vi "E517_Wavegen_Caller.vi"(0 "System no.":i32=1 min=1 step=1, 1 "# Wavegenerators":i32, 2 "Programmatic events":T1(array[ring]), 3 "FastAxisLength":dbl, 5 "error in":errorcluster, 6 "Enabled":bool[](array[boolean])=[FALSE, FALSE, FALSE, FALSE, FALSE, FALSE, FALSE, FALSE], 7 "# WG cycles":i32[](array[numeric]) format="%#.0f", 8 "N":i32=1000, 9 "SIN_P parameters":cluster{"C":dbl, "A":dbl, "O":dbl}={"C"=500.0, "A"=5.0, "O"=0.0} {"O" format="%.6f"; "A" format="%.6f"; "C" format="%.6f"}, 10 "Xo":i32=1, 11 "TriggerVal":i32[](array[numeric])=[0, 1, 2, 4, 5, 6, 8, 9, 10, 11, 12, 14, 15, 16, 18, 19, 20, 21, 22, 24, 25, 26, 28, 29, 30, 31, 32, 34, 35, 36, 38, 39, 40, 41, 42, 44, 45, 46, 48, 49, 50, 51, 52, 54, 55, 56, 58, 59, 60, 61, 62, 64, 65, 66, 68, 69, 70, 71, 72, 74, 75, 76, 78, 79, 80, 81, 82, 84, 85, 86, 88, 89, 90, 91, 92, 94, 95, 96, 98, 99, 100, 101, 102, 104, 105, 106, 108, 109, 110, 111, 112, 114, 115, 116, 118, 119, 120, 121, 122, 124, 125, 126, 128, 129, 130, 131, 132, 134, 135, 136, 138, 139, 140, 141, 142, 144, 145, 146, 148, 149, 150, 151, 152, 154, 155, 156, 158, 159, 160, 161, 162, 164, 165, 166, 168, 169, 170, 171, 172, 174, 175, 176, 178, 179, 180, 181, 182, 184, 185, 186, 188, 189, 190, 191, 192, 194, 195, 196, 198, 199, 200, 201, 202, 204, 205, 206, 208, 209, 210, 211, 212, 214, 215, 216, 218, 219, 220, 221, 222, 224, 225, 226, 228, 229, 230, 231, 232, 234, 235, 236, 238, 239, 240, 241, 242, 244, 245, 246, 248, 249, 250, 251, 252, 254, 255, 256, 258, 259, 260, 261, 262, 264, 265, 266, 268, 269, 270, 271, 272, 274, 275, 276, 278, 279, 280, 281, 282, 284, 285, 286, 288, 289, 290, 291, 292, 294, 295, 296, 298, 299, 300, 301, 302, 304, 305, 306, 308, 309, 310, 311, 312, 314, 315, 316, 318, 319, 320, 321, 322, 324, 325, 326, 328, 329, 330, 331, 332, 334, 335, 336, 338, 339, 340, 341, 342, 344, 345, 346, 348, 349, 350, 351, 352, 354, 355, 356, 358, 359, 360, 361, 362, 364, 365, 366, 368, 369, 370, 371, 372, 374, 375, 376, 378, 379, 380, 381, 382, 384, 385, 386, 388, 389, 390, 391, 392, 394, 395, 396, 398, 399, 400, 401, 402, 404, 405, 406, 408, 409, 410, 411, 412, 414, 415, 416, 418, 419, 420, 421, 422, 424, 425, 426, 428, 429, 430, 431, 432, 434, 435, 436, 438, 439, 440, 441, 442, 444, 445, 446, 448, 449, 450, 451, 452, 454, 455, 456, 458, 459, 460, 461, 462, 464, 465, 466, 468, 469, 470, 471, 472, 474, 475, 476, 478, 479, 480, 481, 482, 484, 485, 486, 488, 489, 490, 491, 492, 494, 495, 496, 498, 499, 500, 501, 502, 504, 505, 506, 508, 509, 510, 511, 512, 514, 515, 516, 518, 519, 520, 521, 522, 524, 525, 526, 528, 529, 530, 531, 532, 534, 535, 536, 538, 539, 540, 541, 542, 544, 545, 546, 548, 549, 550, 551, 552, 554, 555, 556, 558, 559, 560, 561, 562, 564, 565, 566, 568, 569, 570, 571, 572, 574, 575, 576, 578, 579, 580, 581, 582, 584, 585, 586, 588, 589, 590, 591, 592, 594, 595, 596, 598, 599, 600, 601, 602, 604, 605, 606, 608, 609, 610, 611, 612, 614, 615, 616, 618, 619, 620, 621, 622, 624], 12 "Segm.Length":i32=1000, 13 "Append?":bool, 14 "Wavepoint":i32[](array[numeric]), 15 "Switch":i32[](array[numeric])=[0, 1, 2, 4, 5, 6, 8, 9, 10, 11, 12, 14, 15, 16, 18, 19, 20, 21, 22, 24, 25, 26, 28, 29, 30, 31, 32, 34, 35, 36, 38, 39, 40, 41, 42, 44, 45, 46, 48, 49, 50, 51, 52, 54, 55, 56, 58, 59, 60, 61, 62, 64, 65, 66, 68, 69, 70, 71, 72, 74, 75, 76, 78, 79, 80, 81, 82, 84, 85, 86, 88, 89, 90, 91, 92, 94, 95, 96, 98, 99, 100, 101, 102, 104, 105, 106, 108, 109, 110, 111, 112, 114, 115, 116, 118, 119, 120, 121, 122, 124, 125, 126, 128, 129, 130, 131, 132, 134, 135, 136, 138, 139, 140, 141, 142, 144, 145, 146, 148, 149, 150, 151, 152, 154, 155, 156, 158, 159, 160, 161, 162, 164, 165, 166, 168, 169, 170, 171, 172, 174, 175, 176, 178, 179, 180, 181, 182, 184, 185, 186, 188, 189, 190, 191, 192, 194, 195, 196, 198, 199, 200, 201, 202, 204, 205, 206, 208, 209, 210, 211, 212, 214, 215, 216, 218, 219, 220, 221, 222, 224, 225, 226, 228, 229, 230, 231, 232, 234, 235, 236, 238, 239, 240, 241, 242, 244, 245, 246, 248, 249, 250, 251, 252, 254, 255, 256, 258, 259, 260, 261, 262, 264, 265, 266, 268, 269, 270, 271, 272, 274, 275, 276, 278, 279, 280, 281, 282, 284, 285, 286, 288, 289, 290, 291, 292, 294, 295, 296, 298, 299, 300, 301, 302, 304, 305, 306, 308, 309, 310, 311, 312, 314, 315, 316, 318, 319, 320, 321, 322, 324, 325, 326, 328, 329, 330, 331, 332, 334, 335, 336, 338, 339, 340, 341, 342, 344, 345, 346, 348, 349, 350, 351, 352, 354, 355, 356, 358, 359, 360, 361, 362, 364, 365, 366, 368, 369, 370, 371, 372, 374, 375, 376, 378, 379, 380, 381, 382, 384, 385, 386, 388, 389, 390, 391, 392, 394, 395, 396, 398, 399, 400, 401, 402, 404, 405, 406, 408, 409, 410, 411, 412, 414, 415, 416, 418, 419, 420, 421, 422, 424, 425, 426, 428, 429, 430, 431, 432, 434, 435, 436, 438, 439, 440, 441, 442, 444, 445, 446, 448, 449, 450, 451, 452, 454, 455, 456, 458, 459, 460, 461, 462, 464, 465, 466, 468, 469, 470, 471, 472, 474, 475, 476, 478, 479, 480, 481, 482, 484, 485, 486, 488, 489, 490, 491, 492, 494, 495, 496, 498, 499, 500, 501, 502, 504, 505, 506, 508, 509, 510, 511, 512, 514, 515, 516, 518, 519, 520, 521, 522, 524, 525, 526, 528, 529, 530, 531, 532, 534, 535, 536, 538, 539, 540, 541, 542, 544, 545, 546, 548, 549, 550, 551, 552, 554, 555, 556, 558, 559, 560, 561, 562, 564, 565, 566, 568, 569, 570, 571, 572, 574, 575, 576, 578, 579, 580, 581, 582, 584, 585, 586, 588, 589, 590, 591, 592, 594, 595, 596, 598, 599, 600, 601, 602, 604, 605, 606, 608, 609, 610, 611, 612, 614, 615, 616, 618, 619, 620, 621, 622, 624]) -> (16 "Triggerpoints":dbl[][](graph), 17 "Wavetable data":dbl[][](graph), 18 "Recordtable data":dbl[][](graph), 19 "Error out":errorcluster)   [LabVIEW 2011]
doc: "This VI demonstrates how to configure the wave generator, set wave tables, read data recorder tables and set trigger points. The diagram shows how to combine the driver VIs for these tasks. \nThe controls connected to the connector pane exemplify the application. You can modify the connector pane and add controls to meet your requirements. The E517_Wavegen_Example_Caller.vi shows how to call this VI programmatically as a SubVI.\n\nRun E517_Configuration_Setup.vi prior to running this VI.\n\nOn the [Settings] tab you can link wave tables to wave generators if this feature is supported by your controller, adjust wave table and record table rates and configure the wave generator. The current wave generator mode setting (WGO), the actual positions and the servo states are updated continuously.\n \nSelect the desired wave table on the [Wavetables] tab to write a waveform into it or to clean a previously stored waveform. #points in WT shows the actual length of the tables. You can apply controller generated sine waves or host PC generated point-by-point ramp waveforms covering the motion range of the appropriate connected stage. Please consult the Context Help window of the WAV.vi the User Manual of your controller for details on waveform settings. After writing a waveform to the controller all waveforms are read back and displayed automatically. You can read out the wave tables manually, too.\n\nAll further tabs are disabled until you have defined one wave table at least.\n \nConfigure the data recorder on the [Recordtables] tab prior to reading out any data. Each data recorder table must be configured separately by choosing a linked axis and an axis related record option. The contents of the data recorder tables are not read out automatically. Reasonable data is only available if at least one wave generator run has been started since the last power-on / reboot of the controller.\n \nOn the [Triggerpoints] tab you can link axes to triggerlines if this feature is supported by your controller. If you want to output trigger pulses synchronized with the wave generator output, activate the Generator Trigger mode by pressing the Set TWS trigger mode button. The trigger related controls will then be activated. In the matrix you can define the active trigger points for each triggerline. They will be written to the controller's RAM by Set these trigger points. To reset trigger points use Clear all trigger points. In the graphics pane the active trigger points are displayed as bars."
panel:
  in  "LIN Parameters":cluster{"J":dbl, "A":dbl, "O":dbl}={"J"=0.0, "A"=10.0, "O"=0.0}
  out "Number of Triggerlines":i32
  out "SubVI":bool
  out "Running?":bool[](array[boolean])
  in  "Tab Control":T2(tab)
  out "Axes":string[](array[string])
  in  "Recordtable rate":i32=1
  in  "Wavegen":i32[](array[numeric])=[1, 2, 3] format="%#.0f"
  out "# Recordtables":i32
  out "# Wavetables":i32
  out "# Wavegenerators":i32
  out "Servo":bool[](array[boolean])
  in  "Wavetable rate":i32[](array[numeric]) format="%#.0f"
  out "Positions":dbl[](array[numeric])
  out "WGO mode":i32[](array[numeric]) format="%#.0f"
  in  "Start at\nEndpoint":bool[](array[boolean])=[FALSE, FALSE, FALSE, FALSE, FALSE, FALSE, FALSE, FALSE]
  in  "DDL init":bool[](array[boolean])=[FALSE, FALSE, FALSE, FALSE, FALSE, FALSE, FALSE, FALSE]
  in  "DDL enable":bool[](array[boolean])=[FALSE, FALSE, FALSE, FALSE, FALSE, FALSE, FALSE, FALSE]
  in  "GWD?":bool
  out "# points in WT":i32[](array[numeric]) format="%#.0f"
  in  "WCL":bool
  in  "Write sine":bool
  in  "Add?":bool
  in  "Write points":bool
  out "Assigned\nwavegenerator":i32
  in  "Wavetable":u16(ring) items=["1"]
  in  "DRC?":bool
  out "Record option":string[](array[string])
  out "Source ID":string[](array[string])
  in  "DRC":bool
  in  "Record option":u16(ring)=1 items=["Target position of axis "=1, "Current position of axis "=2, "Position error of axis "=3, "Voltage of piezo channel "=7, "Control output of axis "=15, "DAC input of piezo channel "=16]
  in  "Axis":u16(ring) items=["1"]
  in  "Record table":u16(ring) items=["1", "2", "3"]
  in  "N:":i32=1000
  in  "X0:":i32=1
  in  "DRR?":bool
  in  "CTO":bool
  in  "TWC":bool
  in  "TWS":bool
  in  "TWS?":bool
  in  "Axis":u16[](array[ring]) items=["1"]
  in  "Clear error":bool
  in  "Stop":bool
  # "E-517 wave generator, data recorder and trigger setting sample program"
  # "This VI demonstrates how to configure the wave generator, set wavetables, read recordtables and set triggerpoints.\nYou can apply controller generated sine waves or host PC generated point-by-point ramp waveforms.\nRun E517_Configuration_Setup.vi prior to running this VI."
  # "Wavegenerator state:"
  # "Wavetable"
  # "1"
  # "2"
  # "3"
  # "4"
  # "5"
  # "6"
  # "7"
  # "8"
  # "Wavegen"
  # "1"
  # "2"
  # "3"
  # "4"
  # "5"
  # "6"
  # "7"
  # "8"
  # "1"
  # "2"
  # "3"
  # "4"
  # "5"
  # "6"
  # "7"
  # "8"
  # "1black 2red 3green 4cyan 5yelllow 6purple 7orange 8blue"
  # "1"
  # "2"
  # "3"
  # "4"
  # "5"
  # "6"
  # "7"
  # "8"
  # "1black 2red 3green 4cyan 5yelllow 6purple 7orange 8blue"
  # "Trigger"
  # "1"
  # "2"
  # "3"
  # "4"
  # "5"
  # "6"
  # "1black 2red 3green 4blue 5yelllow 6purple"
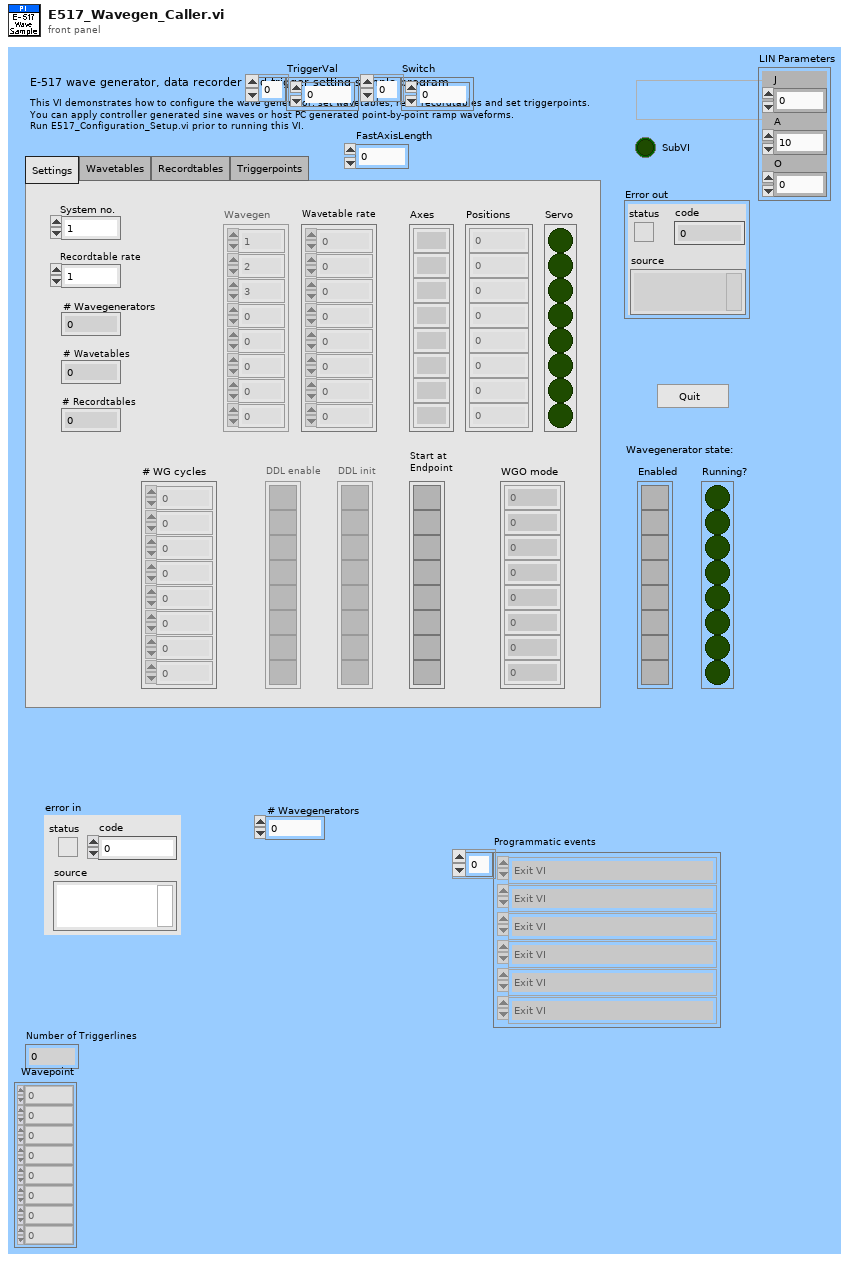
[diagram p1: front panel]
types:
  T1 = enum16{"Exit VI", "Set trigger mode", "Set recordtable rate", "Set wavetable rate", "Write sine", "Read wavetable", "Read recordtable", "Enable/disable wavegen", "Set number of wavegen cycles", "Clear wavetable", "Configure data recorder", "Assign wavetable to wavegen", "Read trigger points", "Set trigger points", "Clear trigger points", "Assign axes to triggerlines", "Write ramp waveform", "Set DDL enable", "Set DDL init", "Set Start at endpoint"}[]
  T2 = enum32{"Settings", "Wavetables", "Recordtables", "Triggerpoints"}
  T3 = enum32{"Page Enabled", "Page Disabled", "Page Disabled & Grayed"}
  T4 = enum16{"Position Distance", "Position Distance & Wait Time", "OnTarget", "MinMax Threshold", "Generator Trigger (TWS)", "Motion Error", "In Motion"}
  T5 = enum16{"Unused", "TriggerStep", "Axis", "TriggerMode", "TriggerDelay", "MinThreshold", "MaxThreshold", "Polarity", "StartThreshold", "StopThreshold"}
  T6 = enum16{"Position Distance", "Position Distance & Wait Time", "OnTarget", "MinMax Threshold", "Generator Trigger (TWS)", "Motion Error", "In Motion"}[]
  T7 = enum16{"Unused", "TriggerStep", "Axis", "TriggerMode", "TriggerDelay", "MinThreshold", "MaxThreshold", "Polarity", "StartThreshold", "StopThreshold"}[]
  T8 = enum16{"Exit VI", "Set trigger mode", "Set recordtable rate", "Set wavetable rate", "Write sine", "Read wavetable", "Read recordtable", "Enable/disable wavegen", "Set number of wavegen cycles", "Clear wavetable", "Configure data recorder", "Assign wavetable to wavegen", "Read trigger points", "Set trigger points", "Clear trigger points", "Assign axes to triggerlines", "Write ramp waveform", "Set DDL enable", "Set DDL init", "Set Start at endpoint"}
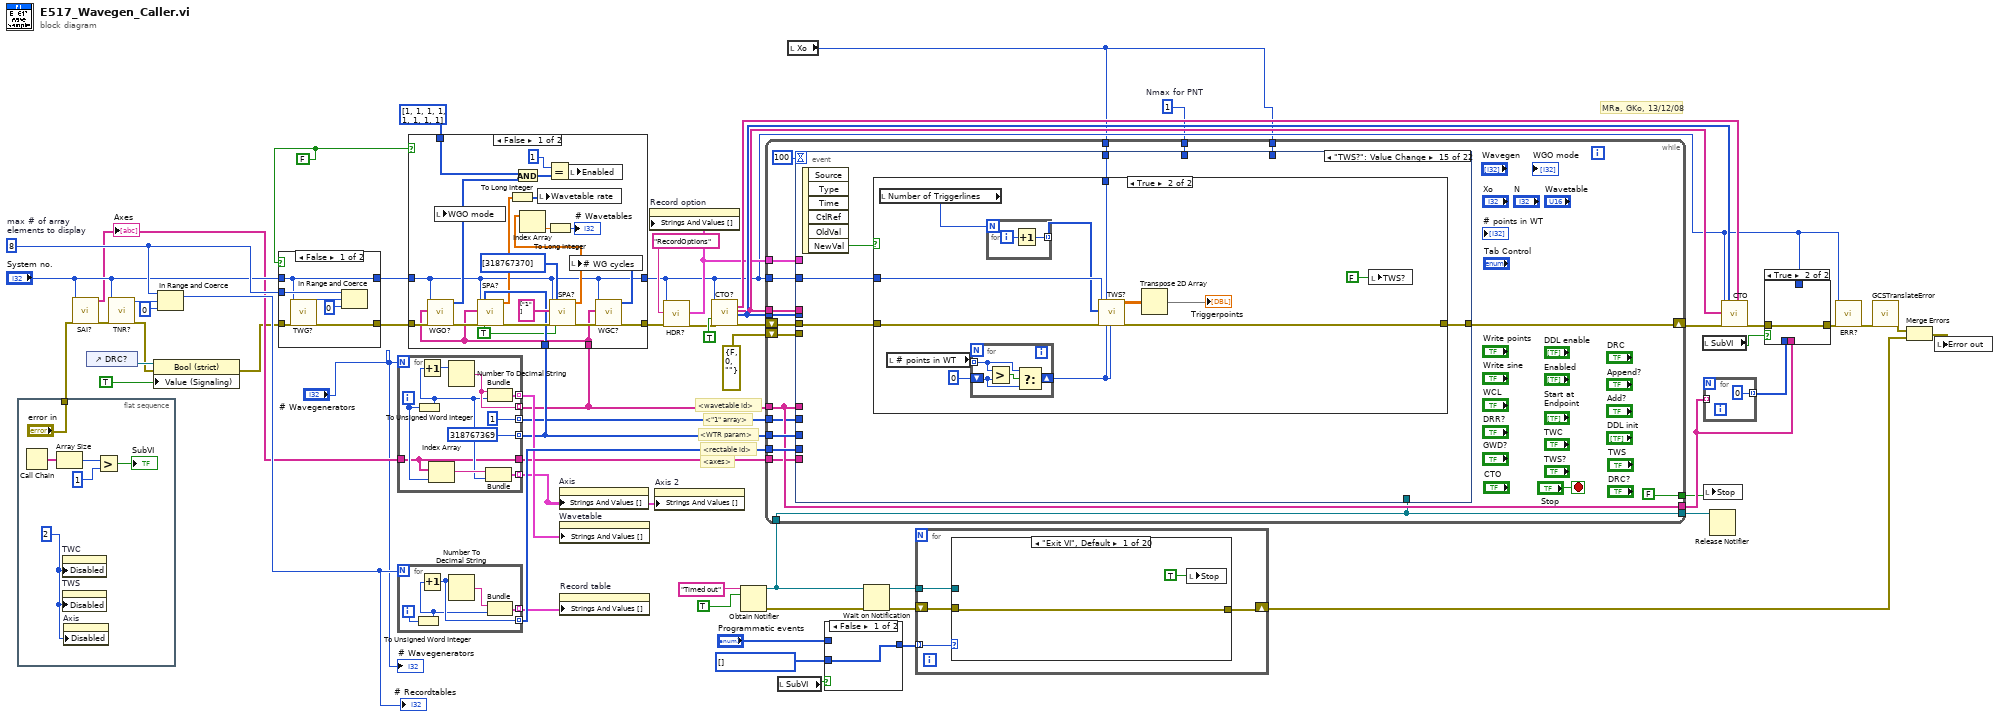
[diagram p0: block diagram]
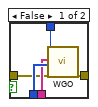
[diagram p2: hidden frame]
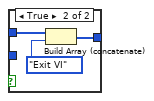
[diagram p5: hidden frame]
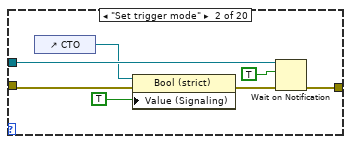
[diagram p6: hidden frame]
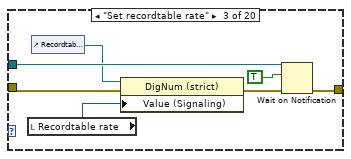
[diagram p7: hidden frame]
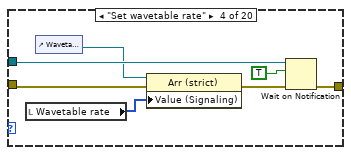
[diagram p8: hidden frame]
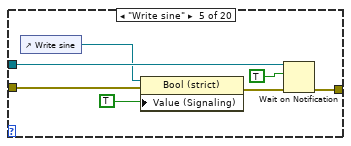
[diagram p9: hidden frame]
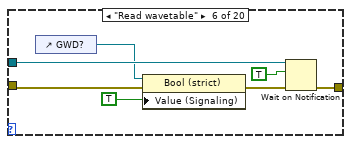
[diagram p10: hidden frame]
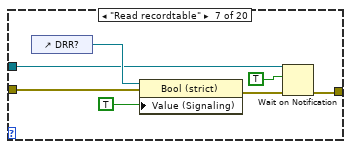
[diagram p11: hidden frame]
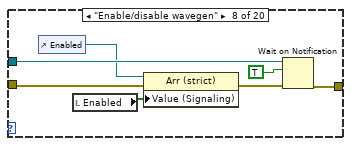
[diagram p12: hidden frame]
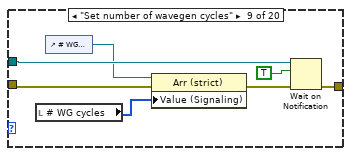
[diagram p13: hidden frame]
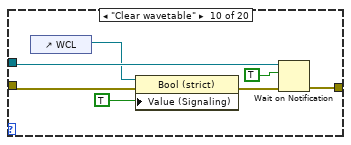
[diagram p14: hidden frame]
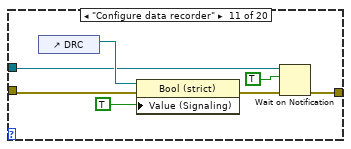
[diagram p15: hidden frame]
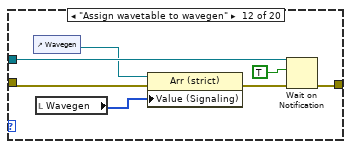
[diagram p16: hidden frame]
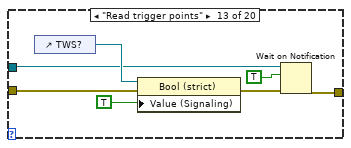
[diagram p17: hidden frame]
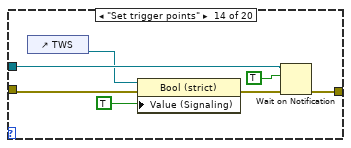
[diagram p18: hidden frame]
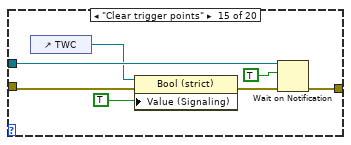
[diagram p19: hidden frame]
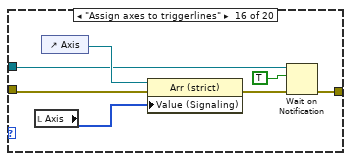
[diagram p20: hidden frame]
diagram:
  w1 = FALSE
  w16 = T1 [] items=["Exit VI", "Set trigger mode", "Set recordtable rate", "Set wavetable rate", "Write sine", "Read wavetable", "Read recordtable", "Enable/disable wavegen", "Set number of wavegen cycles", "Clear wavetable", "Configure data recorder", "Assign wavetable to wavegen", "Read trigger points", "Set trigger points", "Clear trigger points", "Assign axes to triggerlines", "Write ramp waveform", "Set DDL enable", "Set DDL init", "Set Start at endpoint"] ("Programmatic events")
  w4 = 1  # Nmax for PNT
  w13 = 8  # max # of array  elements to display
  # "<axes>"
  # "MRa, GKo, 13/12/08"
  # "<wavetable id>"
  # "<rectable id>"
  # "<\"1\" array>"
  # "<WTR param>"
  n1 = flat-sequence {
    tunnel: ["error in"] -> w20
    frame #0 {
      w61 = u8 2 ("Disabled")
      n2 = Call Chain() -> (call chain=w66:string[])
      n3 = Array Size(array=w66) -> (size(s)=w65:i32)
      n4 = property on="TWC" class="Bool (strict)"("Disabled"=w61) -> ()  [unwired: 2 in, 2 out]
      n5 = property on="TWS" class="Bool (strict)"("Disabled"=w61) -> ()  [unwired: 2 in, 2 out]
      n6 = property on="Axis" class="Arr (strict)"("Disabled"=w61) -> ()  [unwired: 2 in, 2 out]
      n7 = Greater?(x=w65, y=1) -> (0:→"SubVI":bool)
    }
  }
  n8 = call "SAI?.vi"("System no."="System no.", "error in"=w20) -> ("Conn. axes"=w8:string[], "error out"=w51:errorcluster)  [unwired: 3 in, 13 out]
  "Axes" <- w8
  n9 = control-ref of="DRC?"() -> (w48:refnum<vi>)
  n10 = call "TNR?.vi"("System no."="System no.", "error in"=w51) -> ("Number of Rec. tables"=w56:i32, "error out"=w15:errorcluster)  [unwired: 16 out]
  n11 = property class="Bool (strict)"(reference=w48, error in=w15, "Value (Signaling)"=TRUE ("TWC")) -> (error out=w6:errorcluster)  [unwired: 1 out]
  n12 = In Range and Coerce(upper limit=w13, x=w56, lower limit=0) -> (coerced(x)=w10:i32)  [unwired: 1 out]
  "# Recordtables" <- w10
  n13 = case shown="False" w1 {
    tunnel: [w72 w73] -> w14
    tunnel: w6 -> [w71 w73]
    tunnel: w13 -> [w69 _]
    tunnel: "System no." -> [w67 w74]
    tunnel: [w67 w74] -> w11
    frame False {
      n14 = call "TWG?.vi"("System no."=w67, "error in"=w71) -> ("Number of wave generators"=w70:i32, "error out"=w72:errorcluster)  [unwired: 16 out]
      n15 = In Range and Coerce(upper limit=w69, x=w70, lower limit=0) -> ()  [unwired: 2 out]
    }
    frame True {
    }
  }
  n16 = for {
    N: "# Wavegenerators" -> [_]
    tunnel: [w83] -> w58 mode=indexing
    tunnel: [w78] -> w19 mode=indexing
    tunnel: [318767369 ("Numeric")] -> w55 mode=indexing
    tunnel: [1 ("Number of wave generators")] -> w50 mode=indexing
    tunnel: w8 -> [w75]
    tunnel: [w77] -> w5 mode=indexing
    tunnel: [w75] -> w7
    i -> [w80]
    n17 = To Unsigned Word Integer(number=w80) -> (unsigned 16bit integer=w76:u16)
    n18 = Increment(x=w76) -> (x+1=w84:u16)
    n19 = Index Array(array=w75, index=w80) -> (element=w79:string)
    n20 = Number To Decimal String(number=w84) -> (decimal integer string=w78:string)  [unwired: 1 out]
    n21 = Bundle("String"=w79, w76) -> (w77:cluster{"String":string, u16})  [unwired: 1 out]
    n22 = Bundle(w78, w76) -> (w83:cluster{string, u16})  [unwired: 1 out]
  }
  n23 = for {
    N: w10 -> [_]
    tunnel: [w89] -> w59 mode=indexing
    tunnel: [w87] -> w60 mode=indexing
    i -> [w86]
    n24 = To Unsigned Word Integer(number=w86) -> (unsigned 16bit integer=w85:u16)
    n25 = Increment(x=w85) -> (x+1=w87:u16)
    n26 = Number To Decimal String(number=w87) -> (decimal integer string=w88:string)  [unwired: 1 out]
    n27 = Bundle(w88, w85) -> (w89:cluster{string, u16})  [unwired: 1 out]
  }
  n28 = case shown="False" w1 {
    tunnel: w14 -> [w111 w112]
    tunnel: w55 -> [w106 _]
    tunnel: [w105 w112] -> w26
    tunnel: w11 -> [w91 w113]
    tunnel: i32[] [1, 1, 1, 1, 1, 1, 1, 1] ("WGO parameter") -> [w101 _]
    tunnel: [w91 w113] -> w21
    tunnel: w19 -> [w90 _]
    frame False {
      w94 = TRUE ("Parameter no. format \n(Decimal: FALSE)")
      n29 = call "WGO?.vi"("System no."=w91, "Axes to query"=w90, "error in"=w111) -> ("WGO parameter"=w100:i32[], "error out"=w108:errorcluster)  [unwired: 2 in, 13 out]
      n30 = local write "WGO mode"(w100) -> ()
      n31 = call "SPA?.vi"("System no."=w91, "Axes to query"=w90, "error in"=w108, "Parameter no. (hex)"=w106, "Parameter no. format \n(Decimal: FALSE)"=w94) -> ("Parameter value"=w98:dbl[], "error out"=w107:errorcluster)  [unwired: 2 in, 11 out]
      n32 = To Long Integer(number=w98) -> (32bit integer=w99:i32[])
      n33 = And(x=w101, y=w100) -> (x .and. y?=w102:i32[])
      n34 = local write "Wavetable rate"(w99) -> ()
      n35 = Equal?(x=1, y=w102) -> (x = y?=w104:bool[])
      n36 = call "SPA?.vi"("System no."=w91, "Axes to query"=string[] ["1"], "error in"=w107, "Parameter no. (hex)"=u32[] [318767370], "Parameter no. format \n(Decimal: FALSE)"=w94) -> ("Parameter value"=w92:dbl[], "error out"=w110:errorcluster)  [unwired: 2 in, 11 out]
      n37 = Index Array(array=w92) -> (element=w97:dbl)  [unwired: 1 in]
      n38 = To Long Integer(number=w97) -> (32bit integer=→"# Wavetables":i32)
      n39 = local write "Enabled"(w104) -> ()
      n40 = call "WGC?.vi"("System no."=w91, "Axes to query"=w90, "error in"=w110) -> ("Cycles"=w95:i32[], "error out"=w105:errorcluster)  [unwired: 2 in, 13 out]
      n41 = local write "# WG cycles"(w95) -> ()
    }
    frame True {
    }
  }
  n42 = property on="Axis" class="Ring (strict)"("Strings And Values []"=w5) -> ()  [unwired: 2 in, 2 out]
  n43 = property on="Wavetable" class="Ring (strict)"("Strings And Values []"=w58) -> ()  [unwired: 2 in, 2 out]
  n44 = property on="Record table" class="Ring (strict)"("Strings And Values []"=w59) -> ()  [unwired: 2 in, 2 out]
  n45 = property on="Axis 2" class="Ring (strict)"("Strings And Values []"=w5) -> ()  [unwired: 2 in, 2 out]
  n46 = call "HDR?.vi"("System no."=w21, "Section header"="RecordOptions" ("Header"), "error in"=w26) -> ("Enum values"=w23:cluster{"token string":string, i32}[], "error out"=w25:errorcluster)  [unwired: 15 out]
  n47 = property on="Record option" class="Ring (strict)"("Strings And Values []"=w23) -> ()  [unwired: 2 in, 2 out]
  n48 = call "CTO?.vi"("System no."=w21, "All Triggers?"=TRUE, "error in"=w25) -> ("Parameter value"=w41:string[], "TriggerOut to query out"=w39:string[], "CTO parameter ID out"=w40:i32[], "error out"=w47:errorcluster)  [unwired: 2 in, 11 out]
  n49 = Obtain Notifier(name (unnamed)="Timed out", notification data type=TRUE ("GWD?")) -> (notifier out=w30:refnum<notifier>, error out=w33:errorcluster)  [unwired: 2 in, 1 out]
  n50 = local read "SubVI"() -> (w18:bool)
  n51 = local read "Xo"() -> (w3:i32)
  n52 = while {
    tunnel: w21 -> [w123]
    shift-right: [w127] -> w43
    shift-left: w47 -> [w131]
    tunnel: w19 -> [w125]
    tunnel: w60 -> [w129]
    tunnel: w23 -> [w128]
    tunnel: w55 -> [w126]
    tunnel: [w125] -> w44
    shift-left: errorcluster {"status"=FALSE, "code"=0, "source"=""} ("error in") -> [w124]
    tunnel: w50 -> [w122]
    tunnel: w3 -> [w121]
    tunnel: w3 -> [w120]
    tunnel: w4 -> [w119]
    tunnel: w40 -> [w118]
    tunnel: w39 -> [w117]
    tunnel: [FALSE ("Stop")] -> w37
    tunnel: [w115] -> w34
    tunnel: w30 -> [w115]
    tunnel: w7 -> [w114]
    stop <- "Stop" stop-if-true
    n53 = event shown="[14] \"TWS?\": Value Change" {
      selector: _ -> [_ _ _ _ _ _ _ _ _ _ _ _ _ _ _ _ _ _ _ _ _ _]
      dyn-events: _ -> [_ _ _ _ _ _ _ _ _ _ _ _ _ _ _ _ _ _ _ _ _ _]
      timeout: 100 -> [_ _ _ _ _ _ _ _ _ _ _ _ _ _ _ _ _ _ _ _ _ _]
      tunnel: w131 -> [w140 w187 w219 w227 w230 w260 w265 w301 w330 w335 w338 w362 w386 w412 w416 w440 w469 w483 w504 w535 w544 w553]
      tunnel: w123 -> [w144 w185 w217 w223 w229 _ w264 w300 w321 w334 w337 w361 w385 _ w415 w439 w467 w486 w503 _ _ _]
      tunnel: w125 -> [_ _ _ w222 w231 _ w266 w302 w320 w333 w339 _ w387 _ _ _ _ _ w502 _ _ _]
      tunnel: w129 -> [_ _ _ _ _ _ _ w299 _ _ _ w360 _ _ _ _ _ _ _ _ _ _]
      tunnel: w128 -> [_ _ _ _ _ _ _ _ _ _ _ w359 w384 _ _ _ _ _ _ _ _ _]
      tunnel: [w141 w186 w218 w226 w228 w260 w263 w298 w322 w331 w336 w358 w383 w412 w414 w438 w468 w484 w500 w535 w544 w553] -> w127
      tunnel: w126 -> [_ _ _ w221 _ _ _ _ _ _ _ _ _ _ _ _ _ _ _ _ _ _]
      tunnel: w124 -> [w139 _ _ _ _ _ _ _ _ _ _ _ _ _ _ _ _ _ _ _ _ _]
      tunnel: w122 -> [_ _ _ _ _ _ w262 _ _ _ _ _ _ _ _ _ _ _ _ _ _ _]
      tunnel: w121 -> [_ _ _ _ _ _ w261 _ _ _ _ _ _ _ _ _ _ _ _ _ _ _]
      tunnel: w120 -> [_ _ _ _ _ _ _ _ _ _ _ _ _ _ w413 _ _ _ _ _ _ _]
      tunnel: w119 -> [_ _ _ _ _ _ _ _ _ _ _ _ _ _ _ _ _ _ w499 _ _ _]
      tunnel: w118 -> [_ w184 _ _ _ _ _ _ _ _ _ _ _ _ _ _ _ _ _ _ _ _]
      tunnel: w117 -> [_ w183 _ _ _ _ _ _ _ _ _ _ _ _ _ _ _ _ _ _ _ _]
      tunnel: w115 -> [w133 _ _ _ _ _ _ _ _ _ _ _ _ _ _ _ _ _ _ _ _ _]
      tunnel: w114 -> [_ _ _ _ _ _ _ _ _ _ _ w357 _ _ _ _ _ w490 _ _ _ _]
      event Timeout {
        n54 = event-data() -> ()  [unwired: 3 out]
        n55 = Unbundle By Name(w139) -> ("status"=w137:bool)
        n56 = call "ERR?.vi"("System no."=w144, "error in"=w140) -> ("error out"=w135:errorcluster)  [unwired: 17 out]
        n57 = Unbundle By Name(w135) -> ("status"=w138:bool)
        n58 = Not Equal?(x=w138, y=w137) -> (x != y?=w136:bool)
        n59 = case shown="False" w136 {
          tunnel: w135 -> [w145 w147]
          tunnel: [w145 w146] -> w143
          frame False {
          }
          frame True {
            n60 = call "GCSTranslateError.vi"("error in"=w147) -> ("error out"=w146:errorcluster)  [unwired: 18 out]
          }
        }
        n61 = case shown="No Error" w143 {
          selector: w143 -> [w148 w178]
          tunnel: [w149 w179] -> w141
          tunnel: w144 -> [w161 _]
          frame No Error {
            w151 = TRUE  # All axes?
            n62 = local read "# points in WT"() -> (w155:i32[])
            n63 = Greater Than 0?(x=w155) -> (x > 0?=w154:bool[])
            n64 = Or Array Elements(Boolean array=w154) -> (logical OR=w156:bool)
            n65 = call "#9.vi"("System no."=w161, "error in"=w148) -> ("WG running?"=→"Running?":bool[], "error out"=w164:errorcluster)  [unwired: 16 out]
            n66 = Select(t=T3."Page Enabled" ("Page Enabled State"), s=w156, f=T3."Page Disabled & Grayed" ("Page Enabled State")) -> (s? t:f=w159:T3)
            n67 = call "POS?.vi"("System no."=w161, "All axes?"=w151, "error in"=w164) -> ("Position"=→"Positions":dbl[], "error out"=w162:errorcluster)  [unwired: 2 in, 13 out]
            n68 = call "SVO?.vi"("System no."=w161, "All axes?"=w151, "error in"=w162) -> ("Servo status?"=→"Servo":bool[], "error out"=w150:errorcluster)  [unwired: 2 in, 13 out]
            n69 = property on="Tab Control" class="TabCtl (strict)"(error in=w150) -> (error out=w153:errorcluster, "Pages"=w152:refnum<vi>[])  [unwired: 1 in, 1 out]
            n70 = for {
              shift-right: [w171] -> w149
              shift-left: w153 -> [w172]
              tunnel: w152 -> [w170] mode=indexing
              tunnel: w159 -> [w169]
              i -> [w168]
              n71 = Greater?(x=w168, y=1) -> (0:w166:bool)
              n72 = case shown="True" w166 {
                tunnel: w172 -> [w173 w177]
                tunnel: [w173 w176] -> w171
                tunnel: w170 -> [_ w175]
                tunnel: w169 -> [_ w174]
                frame False {
                }
                frame True {
                  n73 = property class="Page"(reference=w175, error in=w177, "Page Enabled State"=w174) -> (error out=w176:errorcluster)  [unwired: 1 out]
                }
              }
            }
          }
          frame Error {
            n74 = Select(t=errorcluster {"status"=FALSE, "code"=0, "source"=""}, s="Clear error", f=w178) -> (s? t:f=w179:errorcluster)
          }
        }
        "Error out" <- w141
        n75 = Unbundle By Name(w141) -> ("status"=w142:bool)
        n76 = property on="Clear error" class="Bool"("Visible"=w142) -> ()  [unwired: 2 in, 2 out]
        n77 = Send Notification(notification=TRUE, notifier=w133) -> ()  [unwired: 1 in, 2 out]
      }
      event "CTO": Value Change {
        n78 = event-data() -> ("NewVal"=w182:bool)  [unwired: 6 out]
        n79 = case shown="True" w182 {
          tunnel: w187 -> [w188 w205]
          tunnel: [w188 w204] -> w186
          tunnel: w185 -> [_ w203]
          tunnel: w184 -> [_ w202]
          tunnel: w183 -> [_ w201]
          frame False {
          }
          frame True {
            w190 = u8 0 ("Disabled")
            # "Not supported"
            n80 = for {
              tunnel: w202 -> [w211] mode=indexing
              tunnel: w201 -> [w207] mode=indexing
              shift-right: [w208] -> w193
              shift-left: string[] [] -> [w209]
              tunnel: T5."TriggerMode" -> [w206]
              n81 = Equal?(x=w211, y=w206) -> (x = y?=w210:bool)
              n82 = case shown="False" w210 {
                tunnel: w209 -> [w212 w215]
                tunnel: [w212 w214] -> w208
                tunnel: w207 -> [_ w213]
                frame False {
                }
                frame True {
                  n83 = Build Array (concatenate)(w215, w213) -> (w214:string[])
                }
              }
            }
            n84 = property on="TWC" class="Bool (strict)"("Disabled"=w190) -> ()  [unwired: 2 in, 2 out]
            n85 = property on="TWS" class="Bool (strict)"("Disabled"=w190) -> ()  [unwired: 2 in, 2 out]
            n86 = Array Size(array=w193) -> (size(s)=w199:i32)
            "Number of Triggerlines" <- w199
            n87 = property on="Axis" class="Arr (strict)"("Disabled"=u8 2) -> ()  [unwired: 2 in, 2 out]
            n88 = Initialize Array(T4."Generator Trigger (TWS)", w199) -> (w198:T6)
            n89 = Initialize Array(T5."TriggerMode", w199) -> (w191:T7)
            n90 = Number To Decimal String(number=w198) -> (decimal integer string=w197:string[])  [unwired: 1 out]
            n91 = call "CTO.vi"("System no."=w203, "TriggerOut to set"=w193, "error in"=w205, "CTO parameter ID"=w191, "Parameter value"=w197) -> ("error out"=w204:errorcluster)  [unwired: 1 in, 13 out]
            n92 = local write "CTO"(FALSE ("CTO")) -> ()
          }
        }
      }
      event "Recordtable rate": Value Change {
        n93 = event-data() -> ()  [unwired: 7 out]
        n94 = call "RTR.vi"("System no."=w217, "Table rate"="Recordtable rate", "error in"=w219) -> ("error out"=w218:errorcluster)  [unwired: 16 out]
      }
      event "Wavetable rate": Value Change {
        n95 = event-data() -> ()  [unwired: 7 out]
        n96 = To Double Precision Float(number="Wavetable rate") -> (double precision float=w224:dbl[])
        n97 = call "SPA.vi"("System no."=w223, "Axis to set"=w222, "Parameter value"=w224, "error in"=w227, "Parameter no. format \n(Decimal: FALSE)"=TRUE ("Parameter no. format \n(Decimal: FALSE)"), "Parameter number (hex)"=w221) -> ("error out"=w226:errorcluster)  [unwired: 4 in, 9 out]
      }
      event "Write sine": Value Change {
        n98 = event-data() -> ("NewVal"=w232:bool)  [unwired: 6 out]
        n99 = case shown="True" w232 {
          tunnel: w230 -> [w233 w236]
          tunnel: [w233 w235] -> w228
          tunnel: w229 -> [_ w240]
          tunnel: w231 -> [_ w241]
          frame False {
          }
          frame True {
            w251 = u16 4 items=["SIN", "POL", "TAN", "PNT", "SIN_P", "LIN", "RAMP"] ("Waveform")
            n100 = local read "Wavetable"() -> (w239:u16)
            n101 = local read "N"() -> (w244:i32)
            n102 = local read "Append?"() -> (w248:bool)
            n103 = local read "Xo"() -> (w246:i32)
            n104 = local read "Add?"() -> (w247:bool)
            n105 = Index Array(array=w241, index=w239) -> (element=w250:string)
            n106 = Build Array(w250) -> (w249:string[])
            n107 = call "WAV.vi"("System no."=w240, "Waveform"=w251, "Affected axes"=w249, "Append? (&)"=w248, "Add? (+)"=w247, "error in"=w236, "Xo"=w246, "N"=w244, "Segment length"="Segm.Length", "SIN_P Parameters"="SIN_P parameters") -> ("error out"=w242:errorcluster)  [unwired: 8 in, 9 out]
            n108 = call "Wait for controller ready.vi"("System no."=w240, "error in"=w242) -> ("error out"=w238:errorcluster)  [unwired: 2 in, 15 out]
            n109 = local read "SubVI"() -> (w234:bool)
            n110 = case shown="False" w234 {
              tunnel: w238 -> [w253 w256]
              tunnel: [w252 w256] -> w235
              frame False {
                n111 = control-ref of="GWD?"() -> (w255:refnum<vi>)
                n112 = property class="Bool (strict)"(reference=w255, error in=w253, "Value (Signaling)"=TRUE ("GWD?")) -> (error out=w252:errorcluster)  [unwired: 1 out]
              }
              frame True {
              }
            }
            n113 = local write "Write sine"(FALSE ("Write sine")) -> ()
          }
        }
      }
      event "Wavetable": Value Change {
        n114 = event-data() -> ("NewVal"=w259:u16)  [unwired: 6 out]
        n115 = local read "Wavegen"() -> (w258:i32[])
        n116 = Index Array(array=w258, index=w259) -> (element=→"Assigned\nwavegenerator":i32)
      }
      event "GWD?": Value Change {
        n117 = event-data() -> ("NewVal"=w267:bool)  [unwired: 6 out]
        n118 = case shown="True" w267 {
          tunnel: w265 -> [w268 w278]
          tunnel: [w268 w269] -> w263
          tunnel: w264 -> [_ w275]
          tunnel: w266 -> [_ w274]
          tunnel: w262 -> [_ w273]
          tunnel: w261 -> [_ w272]
          frame False {
          }
          frame True {
            n119 = call "WAV?.vi"("System no."=w275, "Axes to query"=w274, "Parameter no."=w273, "error in"=w278) -> ("WAV Parameter value"=w276:dbl[], "error out"=w271:errorcluster)  [unwired: 14 out]
            n120 = To Long Integer(number=w276) -> (32bit integer=w277:i32[])
            n121 = local write "# points in WT"(w277) -> ()
            n122 = for {
              tunnel: w275 -> [w285]
              tunnel: w274 -> [w284] mode=indexing
              tunnel: [w283] -> w279 mode=indexing
              shift-right: [w286] -> w269
              shift-left: w271 -> [w287]
              tunnel: w277 -> [w281] mode=indexing
              tunnel: w272 -> [w280]
              n123 = Greater Than 0?(x=w281) -> (x > 0?=w282:bool)
              n124 = case shown="True" w282 {
                tunnel: w287 -> [w289 w296]
                tunnel: [w289 w295] -> w286
                tunnel: w285 -> [_ w294]
                tunnel: w284 -> [_ w293]
                tunnel: [dbl[] [] ("Waveform points") w292] -> w283
                tunnel: w281 -> [_ w291]
                tunnel: w280 -> [_ w290]
                frame False {
                }
                frame True {
                  n125 = call "GWD?.vi"("System no."=w294, "Query axis"=w293, "error in"=w296, "Xo"=w290, "N"=w291) -> ("Waveform points"=w292:dbl[], "error out"=w295:errorcluster)  [unwired: 6 in, 7 out]
                }
              }
            }
            "Wavetable data" <- w279
            n126 = local write "GWD?"(FALSE ("GWD?")) -> ()
          }
        }
      }
      event "DRR?": Value Change {
        n127 = event-data() -> ("NewVal"=w297:bool)  [unwired: 6 out]
        n128 = case shown="True" w297 {
          tunnel: w301 -> [w303 w307]
          tunnel: [w303 w313] -> w298
          tunnel: w300 -> [_ w305]
          tunnel: w302 -> [_ _]
          tunnel: w299 -> [_ w308]
          frame False {
          }
          frame True {
            n129 = call "WGR.vi"("System no."=w305, "error in"=w307) -> ("error out"=w306:errorcluster)  [unwired: 17 out]
            n130 = call "DRR?.vi"("System no."=w305, "Rec. table IDs"=w308, "error in"=w306, "Xo"="X0:", "N"="N:") -> ("Data"=w310:dbl[][], "error out"=w313:errorcluster)  [unwired: 2 in, 11 out]
            n131 = Transpose 2D Array(2D array=w310) -> (transposed array=→"Recordtable data":dbl[][])
            n132 = local write "DRR?"(FALSE ("DRR?")) -> ()
          }
        }
      }
      event "Enabled": Value Change {
        w326 = 1
        n133 = event-data() -> ("NewVal"=w324:bool[])  [unwired: 6 out]
        n134 = Array Size(array=w320) -> (size(s)=w319:i32)
        n135 = local read "WGO mode"() -> (w315:i32[])
        n136 = Initialize Array(1, w319) -> (w316:i32[])
        n137 = Boolean To (0,1)(Boolean=w324) -> (0, 1=w325:i16[])
        n138 = local read "SubVI"() -> (w314:bool)
        n139 = Multiply(x=w325, y=w326) -> (x*y=w328:i32[])
        n140 = Not(x=w326) -> (.not. x?=w327:i32)
        n141 = Select(t=w316, s=w314, f=w315) -> (s? t:f=w317:i32[])
        n142 = And(x=w317, y=w327) -> (x .and. y?=w329:i32[])
        n143 = Or(x=w329, y=w328) -> (x .or. y?=w323:i32[])
        n144 = call "WGO.vi"("System no."=w321, "Affected axes"=w320, "WGO Parameter"=w323, "error in"=w330) -> ("error out"=w322:errorcluster)  [unwired: 6 in, 9 out]
        n145 = local write "WGO mode"(w323) -> ()
      }
      event "# WG cycles": Value Change {
        n146 = event-data() -> ()  [unwired: 7 out]
        n147 = call "WGC.vi"("System no."=w334, "Affected axes"=w333, "Cycles"="# WG cycles", "error in"=w335) -> ("error out"=w331:errorcluster)  [unwired: 15 out]
      }
      event "WCL": Value Change {
        n148 = event-data() -> ("NewVal"=w340:bool)  [unwired: 6 out]
        n149 = case shown="True" w340 {
          tunnel: w338 -> [w341 w351]
          tunnel: [w341 w345] -> w336
          tunnel: w337 -> [_ w350]
          tunnel: w339 -> [_ w349]
          frame False {
          }
          frame True {
            n150 = local read "Wavetable"() -> (w344:u16)
            n151 = Index Array(array=w349, index=w344) -> (element=w348:string)
            n152 = Build Array(w348) -> (w347:string[])
            n153 = call "WCL.vi"("System no."=w350, "WCL axes"=w347, "error in"=w351) -> ("error out"=w346:errorcluster)  [unwired: 6 in, 10 out]
            n154 = local read "SubVI"() -> (w343:bool)
            n155 = case shown="False" w343 {
              tunnel: w346 -> [w353 w356]
              tunnel: [w352 w356] -> w345
              frame False {
                n156 = control-ref of="GWD?"() -> (w355:refnum<vi>)
                n157 = property class="Bool (strict)"(reference=w355, error in=w353, "Value (Signaling)"=TRUE ("GWD?")) -> (error out=w352:errorcluster)  [unwired: 1 out]
              }
              frame True {
              }
            }
            n158 = local write "WCL"(FALSE ("WCL")) -> ()
          }
        }
      }
      event "DRC": Value Change {
        n159 = event-data() -> ("NewVal"=w363:bool)  [unwired: 6 out]
        n160 = case shown="True" w363 {
          tunnel: w362 -> [w364 w377]
          tunnel: [w364 w368] -> w358
          tunnel: w361 -> [_ w374]
          tunnel: w357 -> [_ w376]
          tunnel: w360 -> [_ w373]
          tunnel: w359 -> [_ _]
          frame False {
          }
          frame True {
            # "It's always connected\nwavegen 1 <-> axis 1,\n2 <-> 2, 3 <-> 3, etc."
            n161 = Index Array(array=w376, index="Axis") -> (element=w365:string)
            n162 = Index Array(array=w373, index="Record table") -> (element=w375:u16)
            n163 = call "DRC.vi"("System no."=w374, "Rec. table"=w375, "Rec. option"="Record option", "error in"=w377, "Source ID"=w365) -> ("error out"=w369:errorcluster)  [unwired: 1 in, 13 out]
            n164 = local read "SubVI"() -> (w367:bool)
            n165 = case shown="False" w367 {
              tunnel: w369 -> [w379 w382]
              tunnel: [w378 w382] -> w368
              frame False {
                n166 = control-ref of="DRC?"() -> (w381:refnum<vi>)
                n167 = property class="Bool (strict)"(reference=w381, error in=w379, "Value (Signaling)"=TRUE ("TWC")) -> (error out=w378:errorcluster)  [unwired: 1 out]
              }
              frame True {
              }
            }
            n168 = local write "DRC"(FALSE ("DRC")) -> ()
          }
        }
      }
      event "DRC?": Value Change {
        n169 = event-data() -> ("NewVal"=w388:bool)  [unwired: 6 out]
        n170 = case shown="True" w388 {
          tunnel: w386 -> [w389 w394]
          tunnel: [w389 w391] -> w383
          tunnel: w385 -> [_ w397]
          tunnel: w387 -> [_ _]
          tunnel: w384 -> [_ w395]
          frame False {
          }
          frame True {
            n171 = call "DRC?.vi"("System no."=w397, "error in"=w394) -> ("Rec. option"=w396:i32[], "Source ID"=→"Source ID":string[], "error out"=w391:errorcluster)  [unwired: 2 in, 13 out]
            n172 = for {
              tunnel: w396 -> [w402] mode=indexing
              tunnel: [w401] -> w393 mode=indexing
              tunnel: w395 -> [w398]
              n173 = Array Size(array=w398) -> (size(s)=w400:i32)
              n174 = Decrement(x=w400) -> (x-1=w399:i32)
              n175 = while {
                tunnel: w398 -> [w411] mode=indexing
                tunnel: [w409] -> w401
                tunnel: w402 -> [w408]
                tunnel: w399 -> [w406]
                i -> [w407]
                stop <- w405 stop-if-true
                n176 = Unbundle(w411) -> ("token string"=w409:string, w410:i32)
                n177 = Greater Or Equal?(x=w407, y=w406) -> (x >= y?=w404:bool)
                n178 = Equal?(x=w410, y=w408) -> (x = y?=w403:bool)
                n179 = Or(x=w403, y=w404) -> (x .or. y?=w405:bool)
              }
            }
            "Record option" <- w393
            n180 = local write "DRC?"(FALSE ("DRC?")) -> ()
          }
        }
      }
      event "Wavegen": Value Change {
        # "Not supported by this controller"
        n181 = event-data() -> ()  [unwired: 7 out]
      }
      event "TWS?": Value Change {
        n182 = event-data() -> ("NewVal"=w417:bool)  [unwired: 6 out]
        n183 = case shown="True" w417 {
          tunnel: w416 -> [w418 w430]
          tunnel: [w418 w423] -> w414
          tunnel: w415 -> [_ w429]
          tunnel: w413 -> [_ w421]
          frame False {
          }
          frame True {
            n184 = local read "Number of Triggerlines"() -> (w419:i32)
            n185 = local read "# points in WT"() -> (w428:i32[])
            n186 = for {
              tunnel: w428 -> [w433] mode=indexing
              shift-right: [w435] -> w422
              shift-left: 0 -> [w434]
              n187 = Greater?(x=w433, y=w434) -> (0:w436:bool)
              n188 = Select(t=w433, s=w436, f=w434) -> (s? t:f=w435:i32)
            }
            n189 = for {
              N: w419 -> [_]
              tunnel: [w431] -> w426 mode=indexing
              i -> [w432]
              n190 = Increment(x=w432) -> (x+1=w431:i32)
            }
            n191 = call "TWS?.vi"("System no."=w429, "TriggerOut to query"=w426, "error in"=w430, "Xo"=w421, "N"=w422, "Nmax"=w422) -> ("Data"=w425:dbl[][], "error out"=w423:errorcluster)  [unwired: 1 in, 11 out]
            n192 = Transpose 2D Array(2D array=w425) -> (transposed array=→"Triggerpoints":dbl[][])
            n193 = local write "TWS?"(FALSE ("TWS?")) -> ()
          }
        }
      }
      event "TWS": Value Change {
        n194 = event-data() -> ("NewVal"=w437:bool)  [unwired: 6 out]
        n195 = case shown="True" w437 {
          tunnel: w440 -> [w441 w451]
          tunnel: w439 -> [_ w450]
          tunnel: [w441 w449] -> w438
          frame False {
          }
          frame True {
            n196 = local write "TWS"(FALSE ("TWS")) -> ()
            n197 = for {
              tunnel: w451 -> [w460]
              tunnel: w450 -> [w459]
              tunnel: "TriggerVal" -> [w458] mode=indexing
              tunnel: [w457] -> w444
              tunnel: "Wavepoint" -> [w456] mode=indexing
              tunnel: "Switch" -> [w455] mode=indexing
              n198 = Build Array(w456) -> (w454:i32[])
              n199 = Build Array(w458) -> (w453:i32[])
              n200 = Build Array(w455) -> (w452:i32[])
              n201 = call "TWS.vi"("System no."=w459, "Wavepoint"=w454, "Trigger value"=w453, "Switch"=w452, "error in"=w460) -> ("error out"=w457:errorcluster)  [unwired: 14 out]
            }
            n202 = local read "SubVI"() -> (w447:bool)
            n203 = call "Wait for controller ready.vi"("System no."=w450, "error in"=w444) -> ("error out"=w448:errorcluster)  [unwired: 2 in, 15 out]
            n204 = case shown="True" w447 {
              tunnel: [w464 w465] -> w449
              tunnel: w448 -> [w461 w465]
              frame False {
                n205 = control-ref of="TWS?"() -> (w463:refnum<vi>)
                n206 = property class="Bool (strict)"(reference=w463, error in=w461, "Value (Signaling)"=TRUE ("TWC")) -> (error out=w464:errorcluster)  [unwired: 1 out]
              }
              frame True {
              }
            }
          }
        }
      }
      event "TWC": Value Change {
        n207 = event-data() -> ("NewVal"=w466:bool)  [unwired: 6 out]
        n208 = case shown="True" w466 {
          tunnel: w469 -> [w470 w477]
          tunnel: [w470 w476] -> w468
          tunnel: w467 -> [_ w473]
          frame False {
          }
          frame True {
            n209 = call "TWC.vi"("System no."=w473, "error in"=w477) -> ("error out"=w475:errorcluster)  [unwired: 17 out]
            n210 = call "Wait for controller ready.vi"("System no."=w473, "error in"=w475) -> ("error out"=w474:errorcluster)  [unwired: 2 in, 15 out]
            n211 = local write "TWC"(FALSE ("TWC")) -> ()
            n212 = local read "SubVI"() -> (w472:bool)
            n213 = case shown="True" w472 {
              tunnel: [w479 w482] -> w476
              tunnel: w474 -> [w478 w482]
              frame False {
                n214 = control-ref of="TWS?"() -> (w481:refnum<vi>)
                n215 = property class="Bool (strict)"(reference=w481, error in=w478, "Value (Signaling)"=TRUE ("TWC")) -> (error out=w479:errorcluster)  [unwired: 1 out]
              }
              frame True {
              }
            }
          }
        }
      }
      event "Axis": Value Change {
        # "Not supported by this controller"
        n216 = event-data() -> ()  [unwired: 7 out]
        n217 = for {
          tunnel: "Axis" -> [w498] mode=indexing
          tunnel: w490 -> [w497]
          tunnel: [w494] -> w487 mode=indexing
          tunnel: [w493] -> w485 mode=indexing
          i -> [w496]
          n218 = Increment(x=w496) -> (x+1=w495:i32)
          n219 = Index Array(array=w497, index=w498) -> (element=w493:string)
          n220 = Number To Decimal String(number=w495) -> (decimal integer string=w494:string)  [unwired: 1 out]
        }
        n221 = Array Size(array="Axis") -> (size(s)=w492:i32)
        n222 = Initialize Array(T5."Axis", w492) -> (w488:T7)
        n223 = call "CTO.vi"("System no."=w486, "TriggerOut to set"=w487, "error in"=w483, "CTO parameter ID"=w488, "Parameter value"=w485) -> ("error out"=w484:errorcluster)  [unwired: 1 in, 13 out]
      }
      event "Write points": Value Change {
        n224 = event-data() -> ("NewVal"=w505:bool)  [unwired: 6 out]
        n225 = local read "Wavetable"() -> (w501:u16)
        n226 = case shown="True" w505 {
          tunnel: w504 -> [w506 w512]
          tunnel: [w506 w521] -> w500
          tunnel: w503 -> [_ w517]
          tunnel: w502 -> [_ w528]
          tunnel: w501 -> [_ w522]
          tunnel: w499 -> [_ w516]
          frame False {
          }
          frame True {
            w529 = u16 5 items=["SIN", "POL", "TAN", "PNT", "SIN_P", "LIN", "RAMP"] ("Waveform")
            # "Generate ramp"
            n227 = Bundle By Name(cluster="LIN Parameters", "J"=1.0, "A"="FastAxisLength", "O"=0.0) -> (w510:cluster{"J":dbl, "A":dbl, "O":dbl})
            n228 = local read "N"() -> (w525:i32)
            n229 = local read "Segm.Length"() -> (w515:i32)
            n230 = local read "Append?"() -> (w524:bool)
            n231 = local read "Xo"() -> (w523:i32)
            n232 = local read "Add?"() -> (w520:bool)
            n233 = Index Array(array=w528, index=w522) -> (element=w527:string)
            n234 = Build Array(w527) -> (w526:string[])
            n235 = call "WAV.vi"("System no."=w517, "Waveform"=w529, "Affected axes"=w526, "Append? (&)"=w524, "Add? (+)"=w520, "error in"=w512, "Xo"=w523, "N"=w525, "Nmax for PNT"=w516, "Segment length"=w515, "LIN Parameters"=w510) -> ("error out"=w519:errorcluster)  [unwired: 7 in, 9 out]
            n236 = call "Wait for controller ready.vi"("System no."=w517, "error in"=w519) -> ("error out"=w518:errorcluster)  [unwired: 2 in, 15 out]
            n237 = local read "SubVI"() -> (w514:bool)
            n238 = case shown="True" w514 {
              tunnel: [w532 w534] -> w521
              tunnel: w518 -> [w530 w534]
              frame False {
                n239 = control-ref of="GWD?"() -> (w531:refnum<vi>)
                n240 = property class="Bool (strict)"(reference=w531, error in=w530, "Value (Signaling)"=TRUE ("GWD?")) -> (error out=w532:errorcluster)  [unwired: 1 out]
              }
              frame True {
              }
            }
            n241 = local write "Write points"(FALSE ("Write points")) -> ()
          }
        }
      }
      event "DDL enable": Value Change {
        w541 = 128
        n242 = event-data() -> ("NewVal"=w543:bool[])  [unwired: 6 out]
        n243 = Boolean To (0,1)(Boolean=w543) -> (0, 1=w542:i16[])
        n244 = local read "WGO mode"() -> (w540:i32[])
        n245 = Multiply(x=w542, y=w541) -> (x*y=w538:i32[])
        n246 = Not(x=w541) -> (.not. x?=w539:i32)
        n247 = And(x=w540, y=w539) -> (x .and. y?=w537:i32[])
        n248 = Or(x=w537, y=w538) -> (x .or. y?=w536:i32[])
        n249 = local write "WGO mode"(w536) -> ()
      }
      event "DDL init": Value Change {
        w549 = 64
        n250 = event-data() -> ("NewVal"=w547:bool[])  [unwired: 6 out]
        n251 = local read "WGO mode"() -> (w545:i32[])
        n252 = Boolean To (0,1)(Boolean=w547) -> (0, 1=w548:i16[])
        n253 = Multiply(x=w548, y=w549) -> (x*y=w551:i32[])
        n254 = Not(x=w549) -> (.not. x?=w550:i32)
        n255 = And(x=w545, y=w550) -> (x .and. y?=w552:i32[])
        n256 = Or(x=w552, y=w551) -> (x .or. y?=w546:i32[])
        n257 = local write "WGO mode"(w546) -> ()
      }
      event "Start at\nEndpoint": Value Change {
        w558 = 256
        n258 = event-data() -> ("NewVal"=w554:bool[])  [unwired: 6 out]
        n259 = local read "WGO mode"() -> (w555:i32[])
        n260 = Boolean To (0,1)(Boolean=w554) -> (0, 1=w557:i16[])
        n261 = Multiply(x=w557, y=w558) -> (x*y=w560:i32[])
        n262 = Not(x=w558) -> (.not. x?=w559:i32)
        n263 = And(x=w555, y=w559) -> (x .and. y?=w561:i32[])
        n264 = Or(x=w561, y=w560) -> (x .or. y?=w556:i32[])
        n265 = local write "WGO mode"(w556) -> ()
      }
    }
  }
  n266 = case shown="False" w18 {
    tunnel: [w562 w563] -> w38
    tunnel: "Programmatic events" -> [_ w564]
    tunnel: w16 -> [w562 _]
    frame False {
    }
    frame True {
      n267 = Build Array (concatenate)(w564, T8."Exit VI" ("Enum")) -> (w563:T1)
    }
  }
  n268 = Wait on Notification(notifier=w30, error in (no error)=w33) -> (notifier out=w31:refnum<notifier>, error out=w32:errorcluster)  [unwired: 4 out]
  n269 = for {
    tunnel: w38 -> [w569] mode=indexing
    tunnel: w31 -> [w568]
    shift-right: [w567] -> w28
    shift-left: w32 -> [w566]
    n270 = case shown="\"Exit VI\", Default" w569 {
      tunnel: w568 -> [_ w574 w583 w590 w597 w603 w608 w616 w625 w629 w635 w644 w649 w658 w665 w671 w678 w686 w693 w698]
      tunnel: [w570 w575 w581 w588 w596 w600 w607 w618 w624 w631 w637 w645 w651 w657 w664 w672 w677 w687 w695 w701] -> w567
      tunnel: w566 -> [w570 w572 w582 w589 w595 w602 w609 w617 w623 w630 w638 w646 w652 w659 w666 w674 w681 w688 w694 w702]
      frame "Exit VI", Default {
        n271 = local write "Stop"(TRUE ("Stop")) -> ()
      }
      frame "Set trigger mode" {
        n272 = control-ref of="CTO"() -> (w573:refnum<vi>)
        n273 = property class="Bool (strict)"(reference=w573, error in=w572, "Value (Signaling)"=TRUE ("GWD?")) -> (error out=w577:errorcluster)  [unwired: 1 out]
        n274 = Wait on Notification(notifier=w574, ignore previous (F)=TRUE, error in (no error)=w577) -> (error out=w575:errorcluster)  [unwired: 4 out]
      }
      frame "Set recordtable rate" {
        n275 = local read "Recordtable rate"() -> (w580:i32)
        n276 = control-ref of="Recordtable rate"() -> (w579:refnum<vi>)
        n277 = property class="DigNum (strict)"(reference=w579, error in=w582, "Value (Signaling)"=w580) -> (error out=w585:errorcluster)  [unwired: 1 out]
        n278 = Wait on Notification(notifier=w583, ignore previous (F)=TRUE, error in (no error)=w585) -> (error out=w581:errorcluster)  [unwired: 4 out]
      }
      frame "Set wavetable rate" {
        n279 = local read "Wavetable rate"() -> (w587:i32[])
        n280 = control-ref of="Wavetable rate"() -> (w586:refnum<vi>)
        n281 = property class="Arr (strict)"(reference=w586, error in=w589, "Value (Signaling)"=w587) -> (error out=w592:errorcluster)  [unwired: 1 out]
        n282 = Wait on Notification(notifier=w590, ignore previous (F)=TRUE, error in (no error)=w592) -> (error out=w588:errorcluster)  [unwired: 4 out]
      }
      frame "Write sine" {
        n283 = control-ref of="Write sine"() -> (w594:refnum<vi>)
        n284 = property class="Bool (strict)"(reference=w594, error in=w595, "Value (Signaling)"=TRUE ("GWD?")) -> (error out=w598:errorcluster)  [unwired: 1 out]
        n285 = Wait on Notification(notifier=w597, ignore previous (F)=TRUE, error in (no error)=w598) -> (error out=w596:errorcluster)  [unwired: 4 out]
      }
      frame "Read wavetable" {
        n286 = control-ref of="GWD?"() -> (w601:refnum<vi>)
        n287 = property class="Bool (strict)"(reference=w601, error in=w602, "Value (Signaling)"=TRUE ("GWD?")) -> (error out=w605:errorcluster)  [unwired: 1 out]
        n288 = Wait on Notification(notifier=w603, ignore previous (F)=TRUE, error in (no error)=w605) -> (error out=w600:errorcluster)  [unwired: 4 out]
      }
      frame "Read recordtable" {
        n289 = control-ref of="DRR?"() -> (w610:refnum<vi>)
        n290 = property class="Bool (strict)"(reference=w610, error in=w609, "Value (Signaling)"=TRUE ("GWD?")) -> (error out=w612:errorcluster)  [unwired: 1 out]
        n291 = Wait on Notification(notifier=w608, ignore previous (F)=TRUE, error in (no error)=w612) -> (error out=w607:errorcluster)  [unwired: 4 out]
      }
      frame "Enable/disable wavegen" {
        n292 = control-ref of="Enabled"() -> (w615:refnum<vi>)
        n293 = local read "Enabled"() -> (w614:bool[])
        n294 = property class="Arr (strict)"(reference=w615, error in=w617, "Value (Signaling)"=w614) -> (error out=w620:errorcluster)  [unwired: 1 out]
        n295 = Wait on Notification(notifier=w616, ignore previous (F)=TRUE, error in (no error)=w620) -> (error out=w618:errorcluster)  [unwired: 4 out]
      }
      frame "Set number of wavegen cycles" {
        n296 = local read "# WG cycles"() -> (w621:i32[])
        n297 = control-ref of="# WG cycles"() -> (w622:refnum<vi>)
        n298 = property class="Arr (strict)"(reference=w622, error in=w623, "Value (Signaling)"=w621) -> (error out=w626:errorcluster)  [unwired: 1 out]
        n299 = Wait on Notification(notifier=w625, ignore previous (F)=TRUE, error in (no error)=w626) -> (error out=w624:errorcluster)  [unwired: 4 out]
      }
      frame "Clear wavetable" {
        n300 = control-ref of="WCL"() -> (w628:refnum<vi>)
        n301 = property class="Bool (strict)"(reference=w628, error in=w630, "Value (Signaling)"=TRUE ("GWD?")) -> (error out=w633:errorcluster)  [unwired: 1 out]
        n302 = Wait on Notification(notifier=w629, ignore previous (F)=TRUE, error in (no error)=w633) -> (error out=w631:errorcluster)  [unwired: 4 out]
      }
      frame "Configure data recorder" {
        n303 = control-ref of="DRC"() -> (w636:refnum<vi>)
        n304 = property class="Bool (strict)"(reference=w636, error in=w638, "Value (Signaling)"=TRUE ("GWD?")) -> (error out=w640:errorcluster)  [unwired: 1 out]
        n305 = Wait on Notification(notifier=w635, ignore previous (F)=TRUE, error in (no error)=w640) -> (error out=w637:errorcluster)  [unwired: 4 out]
      }
      frame "Assign wavetable to wavegen" {
        n306 = control-ref of="Wavegen"() -> (w643:refnum<vi>)
        n307 = local read "Wavegen"() -> (w642:i32[])
        n308 = property class="Arr (strict)"(reference=w643, error in=w646, "Value (Signaling)"=w642) -> (error out=w648:errorcluster)  [unwired: 1 out]
        n309 = Wait on Notification(notifier=w644, ignore previous (F)=TRUE, error in (no error)=w648) -> (error out=w645:errorcluster)  [unwired: 4 out]
      }
      frame "Read trigger points" {
        n310 = control-ref of="TWS?"() -> (w650:refnum<vi>)
        n311 = property class="Bool (strict)"(reference=w650, error in=w652, "Value (Signaling)"=TRUE ("GWD?")) -> (error out=w654:errorcluster)  [unwired: 1 out]
        n312 = Wait on Notification(notifier=w649, ignore previous (F)=TRUE, error in (no error)=w654) -> (error out=w651:errorcluster)  [unwired: 4 out]
      }
      frame "Set trigger points" {
        n313 = control-ref of="TWS"() -> (w656:refnum<vi>)
        n314 = property class="Bool (strict)"(reference=w656, error in=w659, "Value (Signaling)"=TRUE ("GWD?")) -> (error out=w661:errorcluster)  [unwired: 1 out]
        n315 = Wait on Notification(notifier=w658, ignore previous (F)=TRUE, error in (no error)=w661) -> (error out=w657:errorcluster)  [unwired: 4 out]
      }
      frame "Clear trigger points" {
        n316 = control-ref of="TWC"() -> (w663:refnum<vi>)
        n317 = property class="Bool (strict)"(reference=w663, error in=w666, "Value (Signaling)"=TRUE ("GWD?")) -> (error out=w668:errorcluster)  [unwired: 1 out]
        n318 = Wait on Notification(notifier=w665, ignore previous (F)=TRUE, error in (no error)=w668) -> (error out=w664:errorcluster)  [unwired: 4 out]
      }
      frame "Assign axes to triggerlines" {
        n319 = local read "Axis"() -> (w670:u16[])
        n320 = control-ref of="Axis"() -> (w673:refnum<vi>)
        n321 = property class="Arr (strict)"(reference=w673, error in=w674, "Value (Signaling)"=w670) -> (error out=w676:errorcluster)  [unwired: 1 out]
        n322 = Wait on Notification(notifier=w671, ignore previous (F)=TRUE, error in (no error)=w676) -> (error out=w672:errorcluster)  [unwired: 4 out]
      }
      frame "Write ramp waveform" {
        n323 = control-ref of="Write points"() -> (w680:refnum<vi>)
        n324 = property class="Bool (strict)"(reference=w680, error in=w681, "Value (Signaling)"=TRUE ("GWD?")) -> (error out=w683:errorcluster)  [unwired: 1 out]
        n325 = Wait on Notification(notifier=w678, ignore previous (F)=TRUE, error in (no error)=w683) -> (error out=w677:errorcluster)  [unwired: 4 out]
      }
      frame "Set DDL enable" {
        n326 = local read "DDL enable"() -> (w684:bool[])
        n327 = control-ref of="DDL enable"() -> (w685:refnum<vi>)
        n328 = property class="Arr (strict)"(reference=w685, error in=w688, "Value (Signaling)"=w684) -> (error out=w690:errorcluster)  [unwired: 1 out]
        n329 = Wait on Notification(notifier=w686, ignore previous (F)=TRUE, error in (no error)=w690) -> (error out=w687:errorcluster)  [unwired: 4 out]
      }
      frame "Set DDL init" {
        n330 = control-ref of="DDL init"() -> (w692:refnum<vi>)
        n331 = local read "DDL init"() -> (w691:bool[])
        n332 = property class="Arr (strict)"(reference=w692, error in=w694, "Value (Signaling)"=w691) -> (error out=w697:errorcluster)  [unwired: 1 out]
        n333 = Wait on Notification(notifier=w693, ignore previous (F)=TRUE, error in (no error)=w697) -> (error out=w695:errorcluster)  [unwired: 4 out]
      }
      frame "Set Start at endpoint" {
        n334 = local read "Start at\nEndpoint"() -> (w699:bool[])
        n335 = control-ref of="Start at\nEndpoint"() -> (w700:refnum<vi>)
        n336 = property class="Arr (strict)"(reference=w700, error in=w702, "Value (Signaling)"=w699) -> (error out=w704:errorcluster)  [unwired: 1 out]
        n337 = Wait on Notification(notifier=w698, ignore previous (F)=TRUE, error in (no error)=w704) -> (error out=w701:errorcluster)  [unwired: 4 out]
      }
    }
  }
  n338 = local read "SubVI"() -> (w9:bool)
  n339 = for {
    tunnel: [0] -> w45 mode=indexing
    tunnel: w44 -> [_] mode=indexing
  }
  n340 = local write "Stop"(w37) -> ()
  n341 = Release Notifier(notifier=w34) -> ()  [unwired: 1 in, 4 out]
  n342 = call "CTO.vi"("System no."=w21, "TriggerOut to set"=w39, "error in"=w43, "CTO parameter ID"=w40, "Parameter value"=w41) -> ("error out"=w42:errorcluster)  [unwired: 1 in, 13 out]
  n343 = case shown="True" w9 {
    tunnel: [w710 w711] -> w53
    tunnel: w45 -> [w709 _]
    tunnel: w44 -> [w708 _]
    tunnel: w42 -> [w707 w711]
    tunnel: w21 -> [w706 _]
    frame False {
      n344 = call "WGO.vi"("System no."=w706, "Affected axes"=w708, "WGO Parameter"=w709, "error in"=w707) -> ("error out"=w710:errorcluster)  [unwired: 6 in, 9 out]
    }
    frame True {
    }
  }
  n345 = call "ERR?.vi"("System no."=w21, "error in"=w53) -> ("error out"=w54:errorcluster)  [unwired: 17 out]
  n346 = call "GCSTranslateError.vi"("error in"=w54) -> ("error out"=w29:errorcluster)  [unwired: 18 out]
  n347 = Merge Errors(w29, w28) -> (w27:errorcluster)
  n348 = local write "Error out"(w27) -> ()
  "# Wavegenerators" <- "# Wavegenerators"
